vi "set_params.vi"(8 "error in (no error)":errorcluster caption="entrée d'erreur (pas d'erreur)", 11 "TruncatedSVD.lvclass 2":refnum<class "TruncatedSVD.lvclass">) -> (0 "error out":errorcluster caption="sortie d'erreur", 3 "TruncatedSVD.lvclass":refnum<class "TruncatedSVD.lvclass">)   [LabVIEW 2020, in "TruncatedSVD.lvclass"]
uses:
  TruncatedSVD.lvclass
  TruncatedSVD.lvclass/TruncatedSVD.ctl
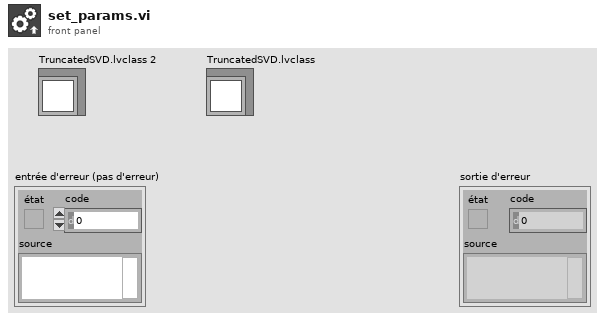
[diagram p1: front panel]
types:
  T1 = typedef "truncated_svd_params.ctl" = cluster{"n_components":dbl, "algorithm":string, "n_iter":dbl, "random_state":dbl, "tol":dbl}
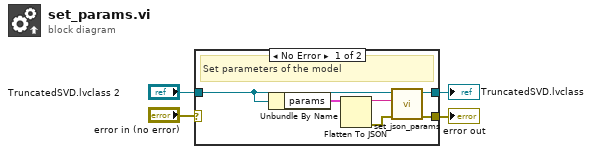
[diagram p0: block diagram]
diagram:
  n1 = case shown="No Error" "error in (no error)" {
    selector: "error in (no error)" -> [_ w12]
    tunnel: [w7 w12] -> w3
    tunnel: [w8 w11] -> w1
    tunnel: "TruncatedSVD.lvclass 2" -> [w5 w11]
    frame No Error {
      # "Set parameters of the model"
      n2 = Unbundle By Name(w5) -> ("params"=w10:T1)
      n3 = Flatten To JSON(anything=w10) -> (JSON string=w9:string, 11:w6:errorcluster)  [unwired: 2 in]
      n4 = call-dynamic "set_json_params.vi"("error in (no error)"=w6, "params"=w9, "Model en entrée"=w5) -> ("error out"=w7:errorcluster, "Model en sortie"=w8:refnum<class "TruncatedSVD.lvclass">)  [unwired: 7 in]
    }
    frame Error {
    }
  }
  "error out" <- w3
  "TruncatedSVD.lvclass" <- w1
